vi "SendToRecord.vi"(8 "error in (no error)":errorcluster, 11 "Record":T1) -> (0 "error out":errorcluster)   [LabVIEW 2015, in "FileHandler.lvlib"]
uses:
  FileHandler.lvlib
  controls/Record.ctl
  <vilib>/addons/Qbus/Qbus.lvclass
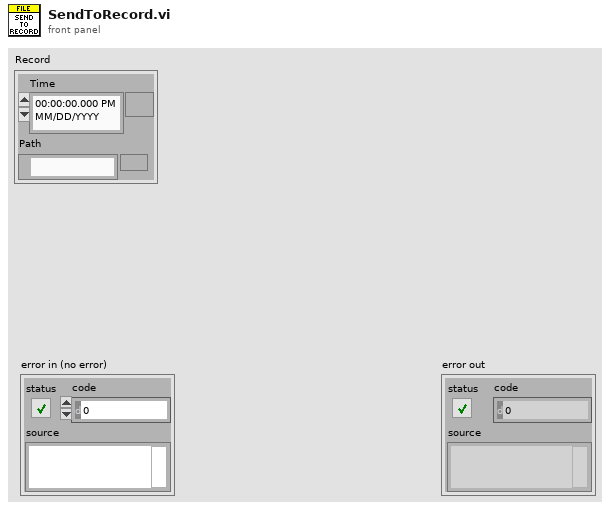
[diagram p1: front panel]
types:
  T1 = typedef "FileHandler.lvlib/Record.ctl" = cluster{"Time":timestamp, "Path":path}
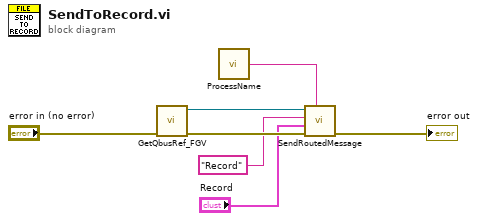
[diagram p0: block diagram]
diagram:
  n1 = call <vilib>:"GetQbusRef_FGV.vi"("error in (no error)"="error in (no error)") -> ("error out"=w6:errorcluster, "Qbus out"=w7:refnum<class "Qbus.lvclass">)  [unwired: 9 in]
  n2 = call "ProcessName.vi"() -> ("process name"=w5:string)  [unwired: 5 in]
  n3 = call <vilib>:"SendRoutedMessage.vi"("listener process"=w5, "error in (no error)"=w6, "message value"="Record", "message name"="Record", "Qbus in"=w7) -> ("error in (no error)"=→"error out":errorcluster)  [unwired: 5 in, 1 out]
